vi "RP convert raw data WFM.vi"(6 "dt":dbl format="%#_6p", 7 "Max Volts":sgl[](array[numeric])=[20.0, 1.0], 8 "Error In":errorcluster, 9 "Signal bits":i32=14, 10 "Format":T1=enum."Digitizer", 11 "data stream":string) -> (0 "Error Out":errorcluster, 1 "element":u32, 2 "phase out":u32[](array[numeric]), 3 "Data out":waveform(sgl)[](array[waveform]))   [LabVIEW 2015]
uses:
  Mode.ctl
  RP ADC to Volts 1D.vi
  RP 32 ADC to Volts 1D.vi
  RP ADC to Volts 2D.vi
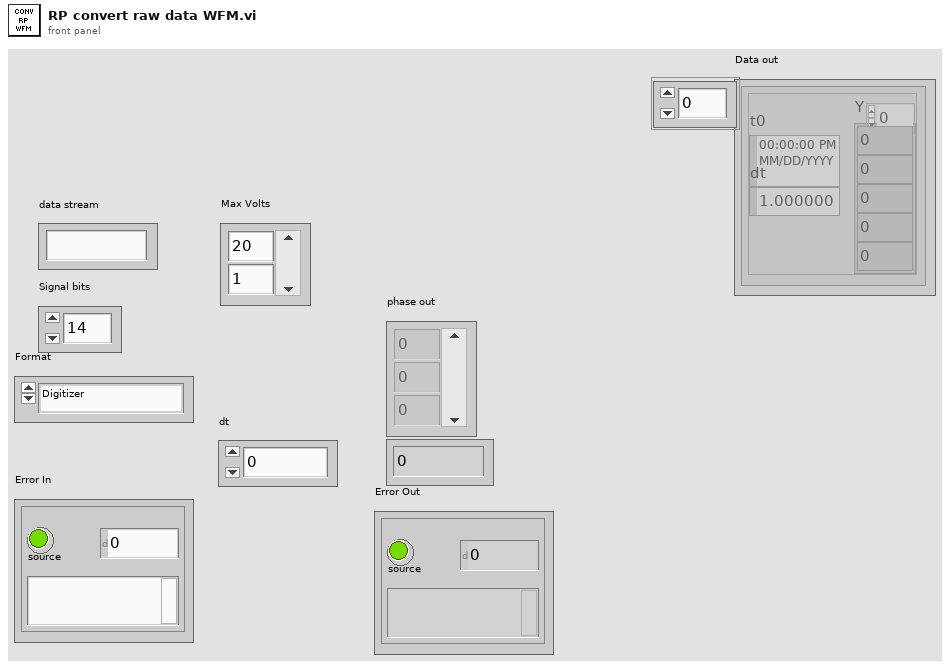
[diagram p1: front panel]
types:
  T1 = typedef "Mode.ctl" = enum16{"Filter", "Lockin test", "Snapshot test", "Digitizer"}
  T2 = enum16{"big-endian, network order", "native, host order", "little-endian"}
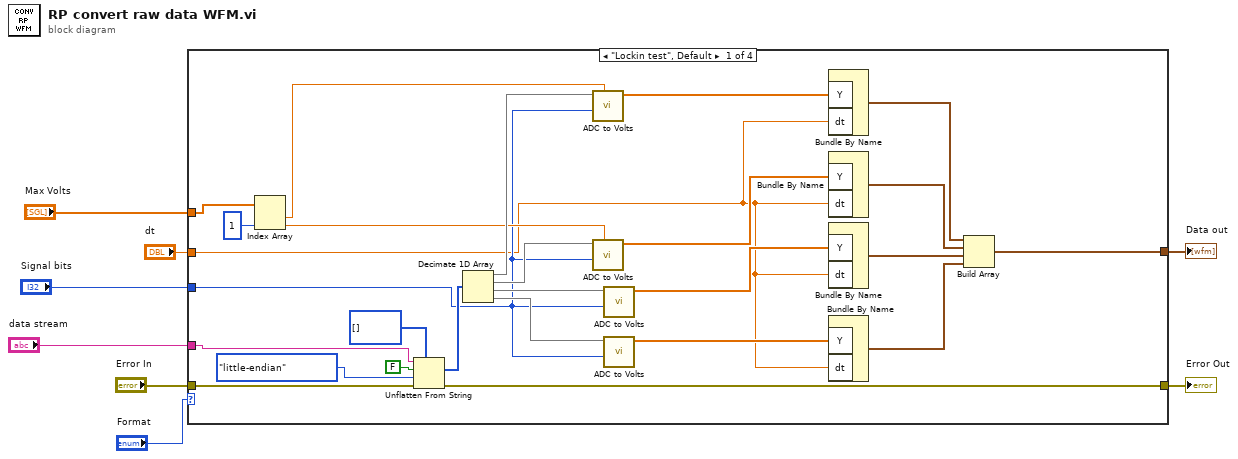
[diagram p0: block diagram]
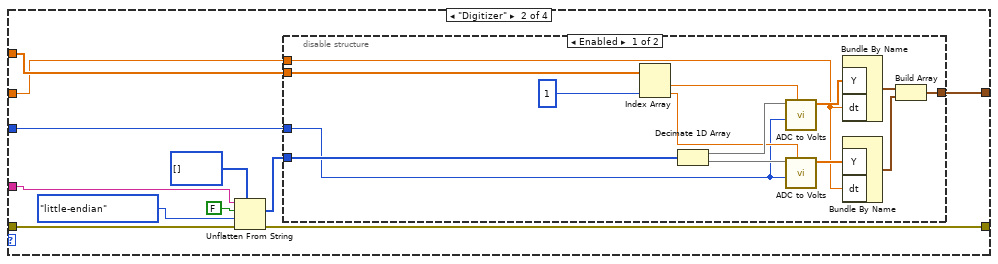
[diagram p2: hidden frame]
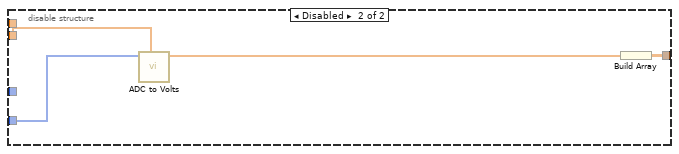
[diagram p3: hidden frame]
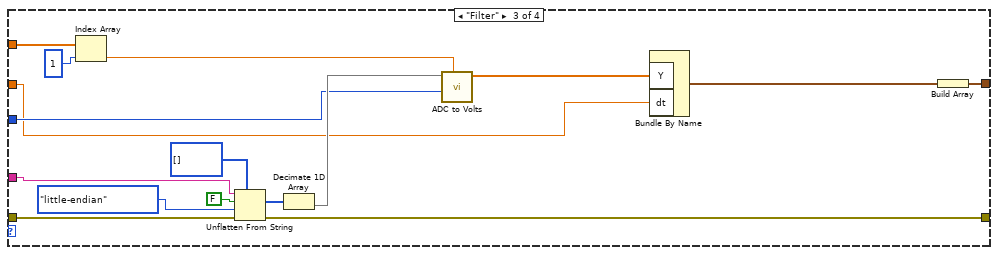
[diagram p4: hidden frame]
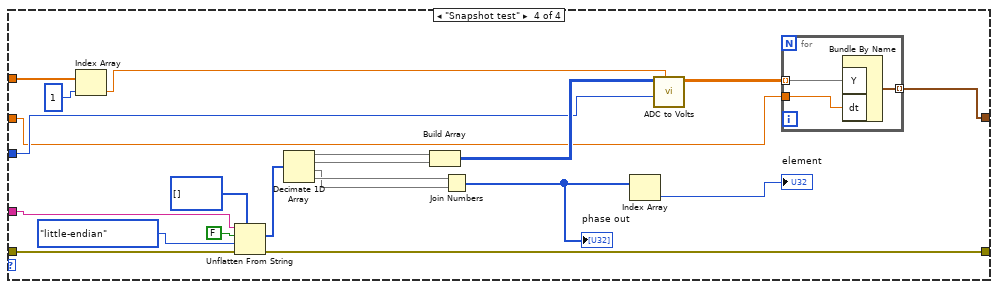
[diagram p5: hidden frame]
diagram:
  n1 = case shown="\"Lockin test\", Default" "Format" {
    tunnel: [w34 w38 w79 w80] -> w1
    tunnel: "Max Volts" -> [w29 w39 w77 w95]
    tunnel: "data stream" -> [w23 w43 w74 w91]
    tunnel: "Error In" -> [w24 w42 w73 w89]
    tunnel: [w22 w37 w70 w88] -> w4
    tunnel: "Signal bits" -> [w18 w36 w67 w83]
    tunnel: "dt" -> [w13 w35 w66 w82]
    frame "Lockin test", Default {
      n2 = Index Array(array=w29, index #2=1 ("index")) -> (element #1=w21:sgl, element #2=w20:sgl)  [unwired: 1 in]
      n3 = Unflatten From String(type=i16[] [], binary string=w23, data includes array or string size? (T)=FALSE, byte order (0:big-endian, network order)=T2."little-endian", error in (no error)=w24) -> (value=w25:i16[], error out=w22:errorcluster)  [unwired: 1 out]
      n4 = Decimate 1D Array(w25) -> (w33:i16[], w32:i16[], w31:i16[], w30:i16[])
      n5 = call-poly "ADC to Volts.vi"("Max Volts"=w21, "Signal bits"=w18, "ADC data"=w33) -> ("Volts"=w17:sgl[])  [unwired: 8 in]
      n6 = call-poly "ADC to Volts.vi"("Max Volts"=w20, "Signal bits"=w18, "ADC data"=w32) -> ("Volts"=w16:sgl[])  [unwired: 8 in]
      n7 = call-poly "ADC to Volts.vi"("Signal bits"=w18, "ADC data"=w31) -> ("Volts"=w15:sgl[])  [unwired: 9 in]
      n8 = call-poly "ADC to Volts.vi"("Signal bits"=w18, "ADC data"=w30) -> ("Volts"=w14:sgl[])  [unwired: 9 in]
      n9 = Bundle By Name("Y"=w17, "dt"=w13) -> (w12:waveform(sgl))  [unwired: 1 in]
      n10 = Bundle By Name("Y"=w16, "dt"=w13) -> (w11:waveform(sgl))  [unwired: 1 in]
      n11 = Bundle By Name("Y"=w15, "dt"=w13) -> (w10:waveform(sgl))  [unwired: 1 in]
      n12 = Bundle By Name("Y"=w14, "dt"=w13) -> (w9:waveform(sgl))  [unwired: 1 in]
      n13 = Build Array(w12, w11, w10, w9) -> (w34:waveform(sgl)[])
    }
    frame "Digitizer" {
      n14 = Unflatten From String(type=i16[] [], binary string=w43, data includes array or string size? (T)=FALSE, byte order (0:big-endian, network order)=T2."little-endian", error in (no error)=w42) -> (value=w40:i16[], error out=w37:errorcluster)  [unwired: 1 out]
      n15 = disable-structure shown="Enabled" {
        disable-tunnel: [w56 w60] -> w38
        disable-tunnel: w40 -> [w59 w62]
        disable-tunnel: w39 -> [w54 w63]
        disable-tunnel: w36 -> [w51 _]
        disable-tunnel: w35 -> [w48 _]
        frame Enabled {
          n16 = Index Array(array=w54, index #2=1 ("index")) -> (element #1=w52:sgl, element #2=w53:sgl)  [unwired: 1 in]
          n17 = Decimate 1D Array(w59) -> (w58:i16[], w57:i16[])
          n18 = call-poly "ADC to Volts.vi"("Max Volts"=w52, "Signal bits"=w51, "ADC data"=w58) -> ("Volts"=w50:sgl[])  [unwired: 8 in]
          n19 = call-poly "ADC to Volts.vi"("Max Volts"=w53, "Signal bits"=w51, "ADC data"=w57) -> ("Volts"=w49:sgl[])  [unwired: 8 in]
          n20 = Bundle By Name("Y"=w50, "dt"=w48) -> (w47:waveform(sgl))  [unwired: 1 in]
          n21 = Bundle By Name("Y"=w49, "dt"=w48) -> (w46:waveform(sgl))  [unwired: 1 in]
          n22 = Build Array(w47, w46) -> (w56:waveform(sgl)[])
        }
        frame Disabled {
          n23 = call-poly "ADC to Volts.vi"("Max Volts"=w63, "ADC data"=w62) -> ("Volts"=w61:sgl[])  [unwired: 9 in]
          n24 = Build Array(w61) -> (w60:sgl[][])
        }
      }
    }
    frame "Filter" {
      n25 = Index Array(array=w77, index=1) -> (element=w69:sgl)
      n26 = Unflatten From String(type=i32[] [], binary string=w74, data includes array or string size? (T)=FALSE, byte order (0:big-endian, network order)=T2."little-endian", error in (no error)=w73) -> (value=w71:i32[], error out=w70:errorcluster)  [unwired: 1 out]
      n27 = Decimate 1D Array(w71) -> (w78:i32[])  [unwired: 1 out]
      n28 = call-poly "ADC to Volts.vi"("Max Volts"=w69, "Signal bits"=w67, "ADC data"=w78) -> ("Volts"=w65:sgl[])  [unwired: 8 in]
      n29 = Bundle By Name("Y"=w65, "dt"=w66) -> (w64:waveform(sgl))  [unwired: 1 in]
      n30 = Build Array(w64) -> (w79:waveform(sgl)[])
    }
    frame "Snapshot test" {
      n31 = Index Array(array=w95, index=1) -> (element=w87:sgl)
      n32 = Unflatten From String(type=i16[] [], binary string=w91, data includes array or string size? (T)=FALSE, byte order (0:big-endian, network order)=T2."little-endian", error in (no error)=w89) -> (value=w90:i16[], error out=w88:errorcluster)  [unwired: 1 out]
      n33 = Decimate 1D Array(w90) -> (w100:i16[], w99:i16[], w97:i16[], w98:i16[])
      n34 = Build Array(w100, w99) -> (w96:i16[][])
      n35 = Join Numbers(hi=w98, lo=w97) -> ((hi.lo)=w85:u32[])
      "phase out" <- w85
      n36 = Index Array(array=w85) -> (element=→"element":u32)  [unwired: 1 in]
      n37 = call-poly "ADC to Volts.vi"("Max Volts"=w87, "Signal bits"=w83, "ADC data"=w96) -> ("Volts"=w81:sgl[][])  [unwired: 8 in]
      n38 = for {
        tunnel: w81 -> [w103] mode=indexing
        tunnel: w82 -> [w102]
        tunnel: [w101] -> w80 mode=indexing
        n39 = Bundle By Name("Y"=w103, "dt"=w102) -> (w101:waveform(sgl))  [unwired: 1 in]
      }
    }
  }
  "Error Out" <- w4
  "Data out" <- w1
